vi "Reset Handshake - Create Resource.vi"() -> (4 "reset handshake item":refnum<k21>)   [LabVIEW 2018, in "Streaming FPGA.lvlib"]
doc: "Creates a handshake item for synchronizing the reset between two clock domains.\n\nOne of the clock domains is the master, the other is the slave. The reset request is processed by the master clock domain. The <B>Reset Handshake - Master</B> VI has a reset input (driven by the reset request) and a reset output. A true on the reset input sets the reset output to true and the output becomes false when the slave clock domain completes the reset cycle. The <B>Reset Handshake - Slave</B> VI has a reset output, and a reset done input. The reset output is set to true for one clock cycle on a reset request received by the master clock domain, and a true on the reset done input signals that the reset cycle completed."
uses:
  <vilib>/rvi/DataTransferAndStorage/Container/Common/niFpgaContainerGetUniqueNameForEmu.vi
  <vilib>/rvi/DataTransferAndStorage/Container/Common/niFpgaContainerSetEmuInfo.vi
  <vilib>/rvi/eio/common/nirviEmuReportErrorAndStop.vi
  <vilib>/rvi/LocalResourceManager/LocalResourceManager.xnode
  Streaming FPGA.lvlib
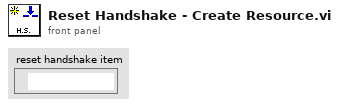
[diagram p1: front panel]
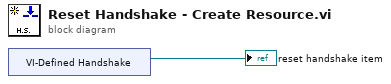
[diagram p0: block diagram]
diagram:
  n1 = xnode "VI-Defined Handshake"() -> ("Handshake Out"=→"reset handshake item":refnum<k21>)
